vi "TRITON_START_COOLDOWN_EXAMPLE.vi"() -> ()   [LabVIEW 2009]
panel:
  out "Connection Open":bool
  in  "Mode":T1(ring)=enum."Immediate"
  in  "Bytes to Read":i32=5000
  in  "IP Address":string
  in  "Remote Port":i32=33576
  in  "Timeout":i32=10000
  in  "Open Connection":bool
  in  "error in (no error)":errorcluster
  out "Cooldown started at:":string
  out "Dewar Pressure Vs Time Plot":cluster{dbl[], dbl[]}(graph)
  out "Dewar [mbar]":dbl
  out "Elapsed Time in Seconds":dbl
  in  "stop":bool
  in  "Pressure to start cooldown\n                  [mbar]":dbl=0.001 format="%#_6e"
  in  "Start Monitoring":bool
  out "error out":errorcluster
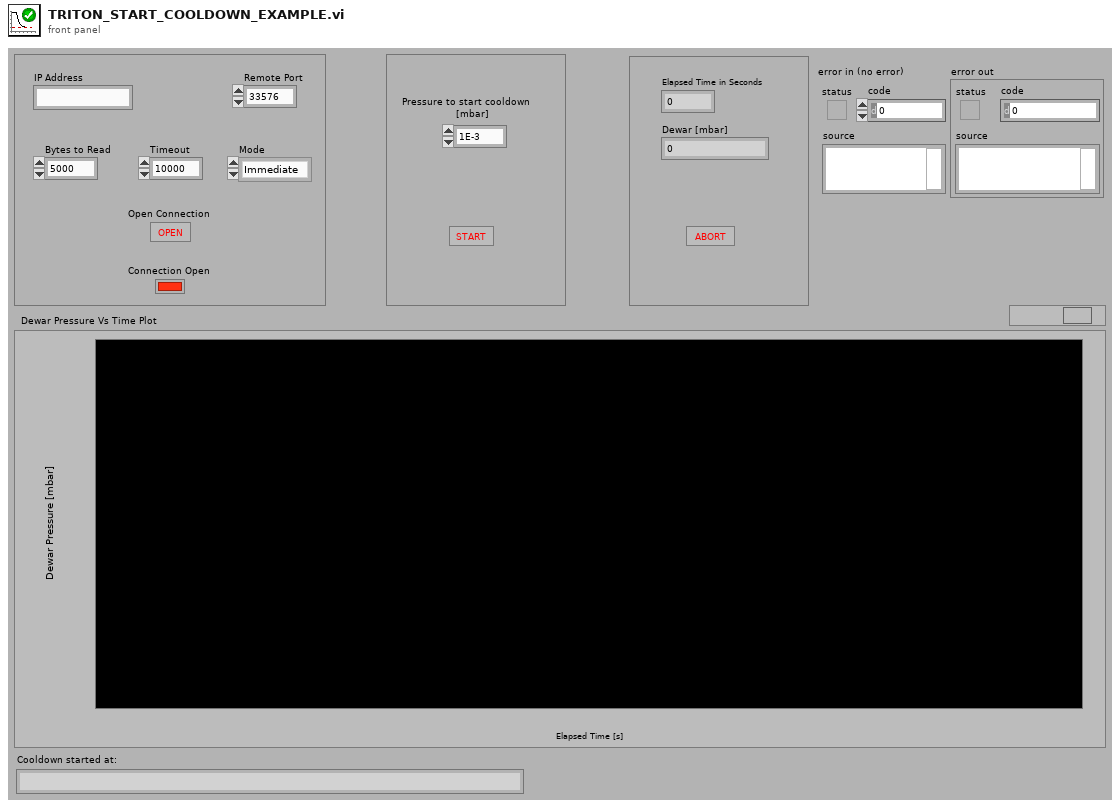
[diagram p1: front panel]
types:
  T1 = enum16{"Standard", "Buffered", "CRLF", "Immediate"}
  T2 = cluster{"Mode":enum16{"Standard", "Buffered", "CRLF", "Immediate"}, "Bytes to Read":i32, "IP Address":string, "Remote Port":i32, "Timeout":i32}
  T3 = cluster{"Mode":enum16{"Standard", "Buffered", "CRLF", "Immediate"}, "Bytes to Read":i32, "IP Address":string, "Remote Port":i32, "Timeout":i32, "connection ID":refnum<k5>}
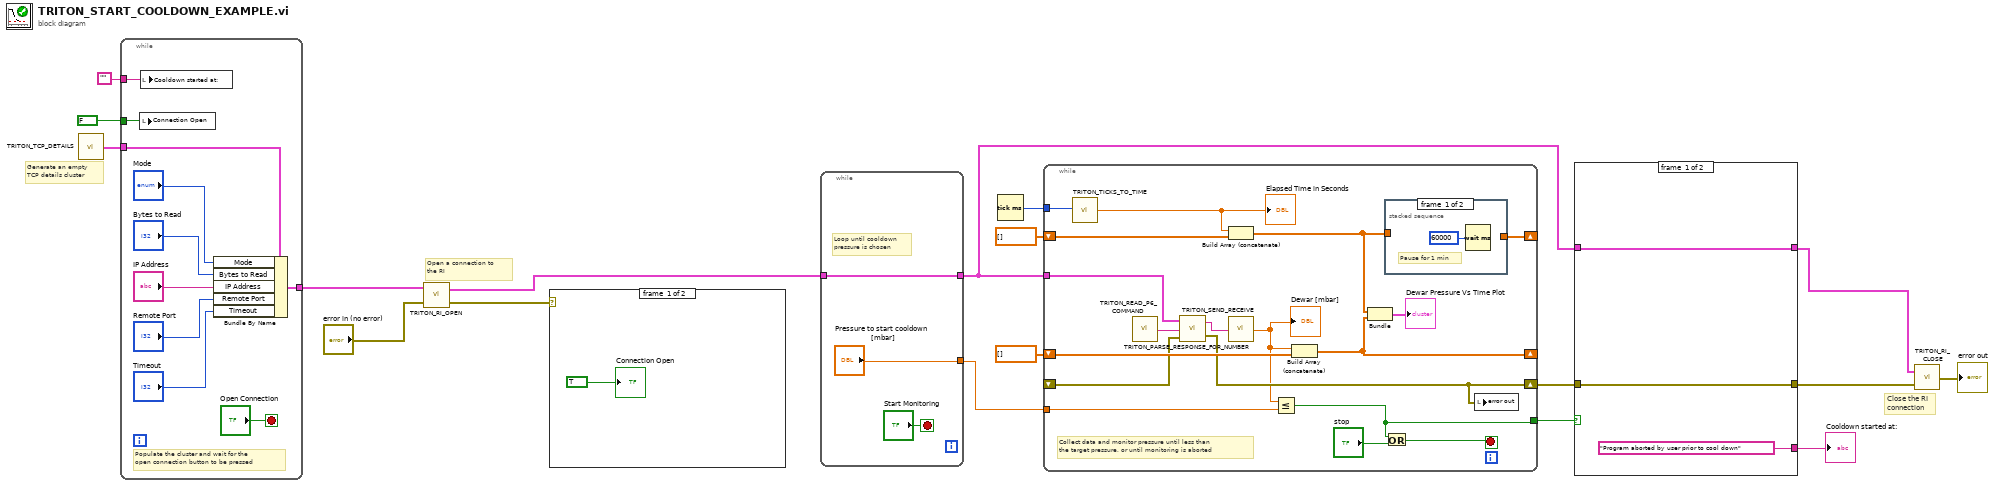
[diagram p0: block diagram]
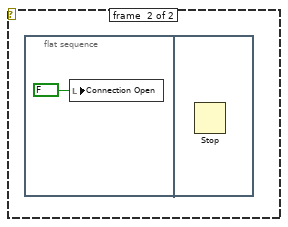
[diagram p2: hidden frame]
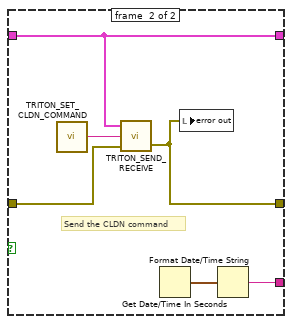
[diagram p3: hidden frame]
diagram:
  # "Open a connection to\nthe RI"
  # "Generate an empty\nTCP details cluster"
  # "Close the RI\nconnection"
  n1 = call "TRITON_TCP_DETAILS.vi"() -> ("Cluster"=w9:T2)
  n2 = while {
    tunnel: w9 -> [w28]
    tunnel: [w21] -> w5
    tunnel: FALSE -> [w20]
    tunnel: "" -> [w19]
    stop <- "Open Connection" stop-if-true
    # "Populate the cluster and wait for the\nopen connection button to be pressed"
    n3 = local write "Connection Open"(w20) -> ()
    n4 = local write "Cooldown started at:"(w19) -> ()
    n5 = Bundle By Name(cluster=w28, "Mode"="Mode", "Bytes to Read"="Bytes to Read", "IP Address"="IP Address", "Remote Port"="Remote Port", "Timeout"="Timeout") -> (w21:T2)
  }
  n6 = call "TRITON_RI_OPEN.vi"("error in (no error)"="error in (no error)", "Cluster"=w5) -> ("error out"=w4:errorcluster, "output cluster"=w3:T3)
  n7 = case shown="Error" w4 {
    frame #0 {
      "Connection Open" <- TRUE
    }
    frame #1 {
      n8 = flat-sequence {
        frame #0 {
          n9 = local write "Connection Open"(FALSE) -> ()
        }
        frame #1 {
          n10 = Stop() -> ()  [unwired: 1 in]
        }
      }
    }
  }
  n11 = while {
    tunnel: ["Pressure to start cooldown\n                  [mbar]"] -> w14
    tunnel: w3 -> [w31]
    tunnel: [w31] -> w2
    stop <- "Start Monitoring" stop-if-true
    # "Loop until cooldown\npressure is chosen"
  }
  n12 = Tick Count (ms)() -> (millisecond timer value=w17:u32)
  n13 = while {
    tunnel: w17 -> [w51]
    shift-right: [w48] -> _
    shift-left: dbl[] [] -> [w49]
    shift-right: [w44] -> _
    shift-left: dbl[] [] -> [w45]
    tunnel: w14 -> [w39]
    shift-right: [w40] -> w11
    shift-left: _ -> [w41]
    tunnel: [w36] -> w13
    tunnel: w2 -> [w35]
    stop <- w38 stop-if-true
    # "Collect data and monitor pressure until less than\nthe target pressure, or until monitoring is aborted"
    n14 = call "TRITON_TICKS_TO_TIME.vi"("Initial millisecond timer value"=w51) -> ("Elapsed Time in Seconds"=w50:dbl)
    "Elapsed Time in Seconds" <- w50
    n15 = call "TRITON_READ_P6_COMMAND.vi"() -> ("Pressures Command String"=w47:string)  [unwired: 1 in]
    n16 = call "TRITON_SEND_RECEIVE.vi"("error in (no error)"=w41, "Command String"=w47, "Communication Cluster"=w35) -> ("error out"=w40:errorcluster, "Response String"=w46:string)
    n17 = Build Array (concatenate)(w50, w49) -> (w43:dbl[])
    n18 = call "TRITON_PARSE_RESPONSE_FOR_NUMBER.vi"("Input String"=w46) -> ("Output"=w34:dbl)
    "Dewar [mbar]" <- w34
    n19 = Less Or Equal?(x=w34, y=w39) -> (x <= y?=w36:bool)
    n20 = Build Array (concatenate)(w34, w45) -> (w44:dbl[])
    n21 = Bundle(w43, w44) -> (→"Dewar Pressure Vs Time Plot":cluster{dbl[], dbl[]})  [unwired: 1 in]
    n22 = stacked-sequence {
      tunnel: w43 -> [_ w53]
      tunnel: [_ w53] -> w48
      frame #0 {
        # "Pause for 1 min"
        n23 = Wait (ms)(milliseconds to wait=u32 60000) -> ()  [unwired: 1 out]
      }
      frame #1 {
      }
    }
    n24 = Or(x=w36, y="stop") -> (x .or. y?=w38:bool)
    n25 = local write "error out"(w40) -> ()
  }
  n26 = case shown="True" w13 {
    tunnel: ["Program aborted by user prior to cool down" ("date/time string") w60] -> w12
    tunnel: w11 -> [w55 w59]
    tunnel: [w55 w58] -> w10
    tunnel: w2 -> [w54 w57]
    tunnel: [w54 w57] -> w1
    frame #0 {
    }
    frame #1 {
      # "Send the CLDN command"
      n27 = call "TRITON_SET_CLDN_COMMAND.vi"() -> ("Command String"=w62:string)  [unwired: 1 in]
      n28 = call "TRITON_SEND_RECEIVE.vi"("error in (no error)"=w59, "Command String"=w62, "Communication Cluster"=w57) -> ("error out"=w58:errorcluster)  [unwired: 1 out]
      n29 = Get Date/Time In Seconds() -> (seconds since 1Jan1904=w61:timestamp)
      n30 = local write "error out"(w58) -> ()
      n31 = Format Date/Time String(seconds (now)=w61) -> (date/time string=w60:string)  [unwired: 2 in]
    }
  }
  "Cooldown started at:" <- w12
  n32 = call "TRITON_RI_CLOSE.vi"("error in (no error)"=w10, "Communication Cluster"=w1) -> ("error out"=→"error out":errorcluster)
